vi "Send Launch Nested Panel Message.vi"(4 "Auto-stop? (T)":bool=TRUE, 6 "timeout in ms (-1)":i32=-1, 7 "Priority":T1=enum."Normal" caption="Message Priority (Normal)", 8 "error in (no error)":errorcluster, 9 "Panel":refnum<class "Panel.lvclass">, 10 "Nested Panel Actor":refnum<class "Panel Actor.lvclass">, 11 "Message Enqueuer in":refnum<class "Message Enqueuer.lvclass">) -> (0 "error out":errorcluster, 2 "Nested Actor's Enqueuer":refnum<class "Message Enqueuer.lvclass">)   [LabVIEW 2023, in "Panel Actor.lvlib" / "Launch Nested Panel Message Msg.lvclass"]
doc: "Sends the <b>Launch Nested Panel Message Msg.lvclass</b> message.\n\nThis message will call <b>Launch Nested Panel Message.vi</b> on the <b>Panel Actor.lvlib:Panel Actor.lvclass</b> actor.\n\n<b>Launch Nested Panel Message.vi Description</b>"
uses:
  Launch Nested Panel Message Msg.lvclass
  builds/Framework/Actor Framework.lvlibp/1abvi3w/vi.lib/ActorFramework/Message Enqueuer/Message Enqueuer.lvclass
  builds/Framework/Actor Framework.lvlibp/1abvi3w/vi.lib/ActorFramework/Message Enqueuer/Message Priority.ctl
  Library/Panel Actor.lvclass
  Panel/Panel/Panel.lvclass
  Launch Nested Panel Message Msg.lvclass/Launch Nested Panel Message Msg.ctl
  C:/Users/Public/Documents/Development/builds/Framework/Actor Framework.lvlibp/1abvi3w/vi.lib/ActorFramework/Message/Message.lvclass
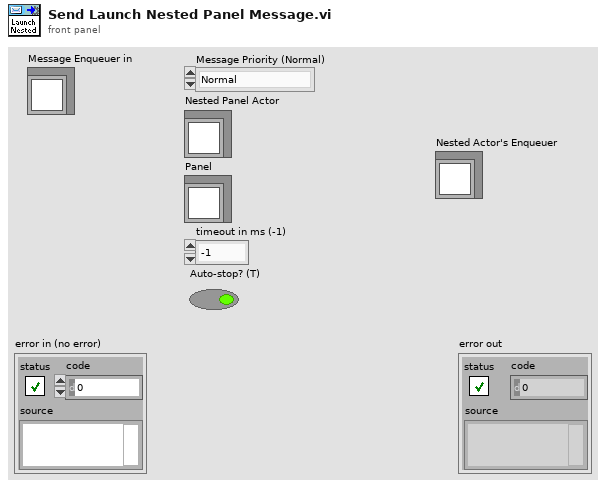
[diagram p1: front panel]
types:
  T1 = typedef "Actor Framework.lvlibp/Message Enqueuer.lvclass/Message Priority.ctl" = enum16{"Low", "Normal", "High"}
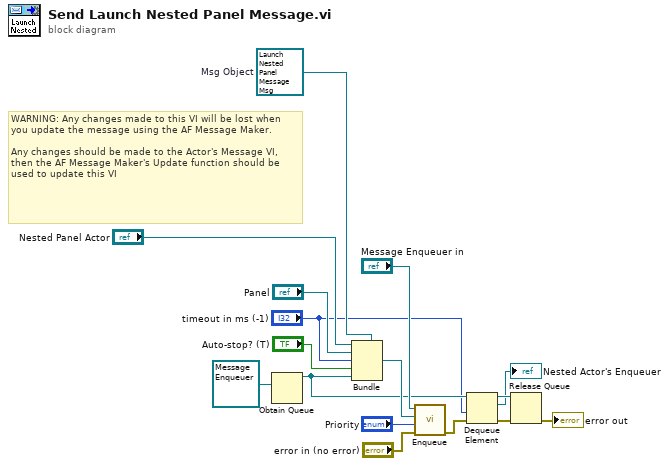
[diagram p0: block diagram]
diagram:
  w13 = refnum<class "Launch Nested Panel Message Msg.lvclass"> refnum  # Msg Object
  # "WARNING: Any changes made to this VI will be lost when you update the message using the AF Message Maker.\n\nAny changes should be made to the Actor's Message VI, then the AF Message Maker's Update function should be used to update this VI"
  n1 = Obtain Queue(element data type=refnum<class "Message Enqueuer.lvclass"> refnum ("Message Enqueuer out")) -> (queue out=w7:refnum<queue>)  [unwired: 4 in, 2 out]
  n2 = Bundle(cluster=w13, "Nested Panel Actor", "Panel", "timeout in ms (-1)", "Auto-stop? (T)", w7) -> (w10:refnum<class "Launch Nested Panel Message Msg.lvclass">)
  n3 = call "Enqueue.vi"("error in (no error)"="error in (no error)", "Message Priority (Normal)"="Priority", "Message"=w10, "Message Enqueuer in"="Message Enqueuer in") -> ("error out"=w4:errorcluster)  [unwired: 6 in, 1 out]
  n4 = Dequeue Element(queue=w7, timeout in ms (-1)="timeout in ms (-1)", error in (no error)=w4) -> (queue out=w6:refnum<queue>, element=→"Nested Actor's Enqueuer":refnum<class "Message Enqueuer.lvclass">, error out=w3:errorcluster)  [unwired: 1 out]
  n5 = Release Queue(queue=w6, error in (no error)=w3) -> (error out=→"error out":errorcluster)  [unwired: 1 in, 2 out]
